vi "uTTA_Main.vi"() -> ()   [LabVIEW 2021]
uses:
  uTTA_Device_Driver/uTTA_Controls/CTL_uTTA_MeasurementStates.ctl
  uTTA_Device_Driver/uTTA_Controls/CTL_uTTA_TSP_Calibration.ctl
  uTTA_Device_Driver/uTTA_Controls/CTL_uTTA_TSP_CalStatus.ctl
  <vilib>/Utility/miscctls.llb/LVPointTypeDef.ctl
  uTTA_Device_Driver/uTTA_Controls/CTL_uTTA_PGA_Gain.ctl
  uTTA_Device_Driver/uTTA_Controls/CTL_uTTA_OperatingMode.ctl
  uTTA_Device_Driver/uTTA_Controls/CTL_uTTA_AnalogParameter.ctl
  <vilib>/Utility/error.llb/DialogType.ctl
  uTTA_Device_Driver/uTTA_SubVi/Serial_Port/uTTA_GV_Serial_Monitor.vi
panel:
  out "Progress / [%]":T1(slide)={"Numeric"=0.0, "Numeric"=3.7741935483870965, "Numeric"=2.3870967741935485} scale=0.0..100.0
  out "uTTA_CalData":T2(array[cluster])
  out "ADC Overrange":bool[](array[boolean])
  out "Heating Power":dbl format="%#_3pW"
  out "Total Runtime":timestamp=timestamp(-3599.4283056259155 s since 1904-01-01) format="%<%H:%M:%S>T"
  out "Measurement Started":timestamp=timestamp(3793474800.1504135 s since 1904-01-01) format="%<%X>T"
  out "Diode Voltages":T3(graph)
  out "Current & Temp":T4(graph)
  in  "Tab Control":T5(tab)
  out "ADC1L_Range":dbl caption="Lower Limit" format="%.2pV"
  out "ADC1H_Range":dbl caption="Upper Limit" format="%.2pV"
  in  "CH1-2 Offset":dbl(slide)=-0.4 scale=-2.5..2.5 scale format="%.2pV"
  out "ADC0H_Range1":dbl caption="Upper Limit" format="%.2pV"
  out "ADC0L_Range1":dbl caption="Lower Limit" format="%.2pV"
  out "ADC0H_Range":dbl caption="Upper Limit" format="%.2pV"
  out "ADC0L_Range":dbl caption="Lower Limit" format="%.2pV"
  in  "CH0 Offset":dbl(slide)=-0.63 scale=-2.5..2.5 scale format="%.2pV"
  in  "Sense Current":dbl(slide)=0.01 caption="CH0" min=0.0 max=0.011 step=0.0001 scale=0.0..0.011 scale format="%.1pA"
  in  "µTTA Port":refnum<visa-resource-name>="COM3"
  in  "Connect":bool
  in  "Disconnect":bool
  in  "Calibration File":path
  in  "Cooling 2":dbl=5400.0 caption="Cooling" min=60.0 max=21600.0 step=1.0 format="%#_g s"
  in  "Heating 2":dbl=5400.0 caption="Heating" min=0.0 max=10800.0 step=1.0 format="%#_g s"
  in  "Preheating":dbl=60.0 min=30.0 max=21600.0 step=1.0 format="%#_g s"
  in  "Cooling":u16(ring)=3 items=["PGA = 0", "PGA = 1", "PGA = 2", "PGA = 3"]
  in  "Heating":u16(ring) items=["PGA = 0", "PGA = 1", "PGA = 2", "PGA = 3"]
  in  "Channel Names":u16[](array[ring])=[0, 0, 0] items=["OFF", "DUMMY1", "DUMMY2", "DUMMY3", "BUZ11", "IRF1010N", "IRF1010N_M", "IRF1010N_L", "IRF1010N_R", "IRFZ44N_M", "IRFZ44N_L", "IRFZ44N_R"]
  in  "Measurement Name":string
  in  "Start":bool
  in  "Stop":bool
  in  "Test Mode":bool
  out "Measurement State":T6=enum."Cooling" caption="uTTA State"
  out "GUI State":string="EXIT"
  in  "FileManager":bool
  out "Files in Flash Memory":string[](array[string])
  in  "Autoscroll":bool
  out "Serial Monitor OUT":string
  in  "Serial Monitor":bool
  in  "Gatedriver Power":bool
  in  "Main Power supply":bool
  in  "Gatedriver":bool
  out "RunTime Error":errorcluster
  out "Exit Error":errorcluster
  out "Device Info":string
  in  "Refresh_CAL":bool
  in  "Cal_Manager":bool
  out "TSP_Channels":T7 {"Offset" format="%.3pV"; "Lin. Gain" format="%#.4pV/K"; "Quad. Gain" format="%.5pV/K²"}
  # "Measurement\nRange"
  # "Measurement Range\nHEATING        COOLING"
  # "Channel Offset"
  # "Sense Current"
  # "T I M I N G"
  # "PGA"
  # "CH0: Driver"
  # "Channel\nNames"
  # "CH1: Monitor1"
  # "CH2: Monitor 2"
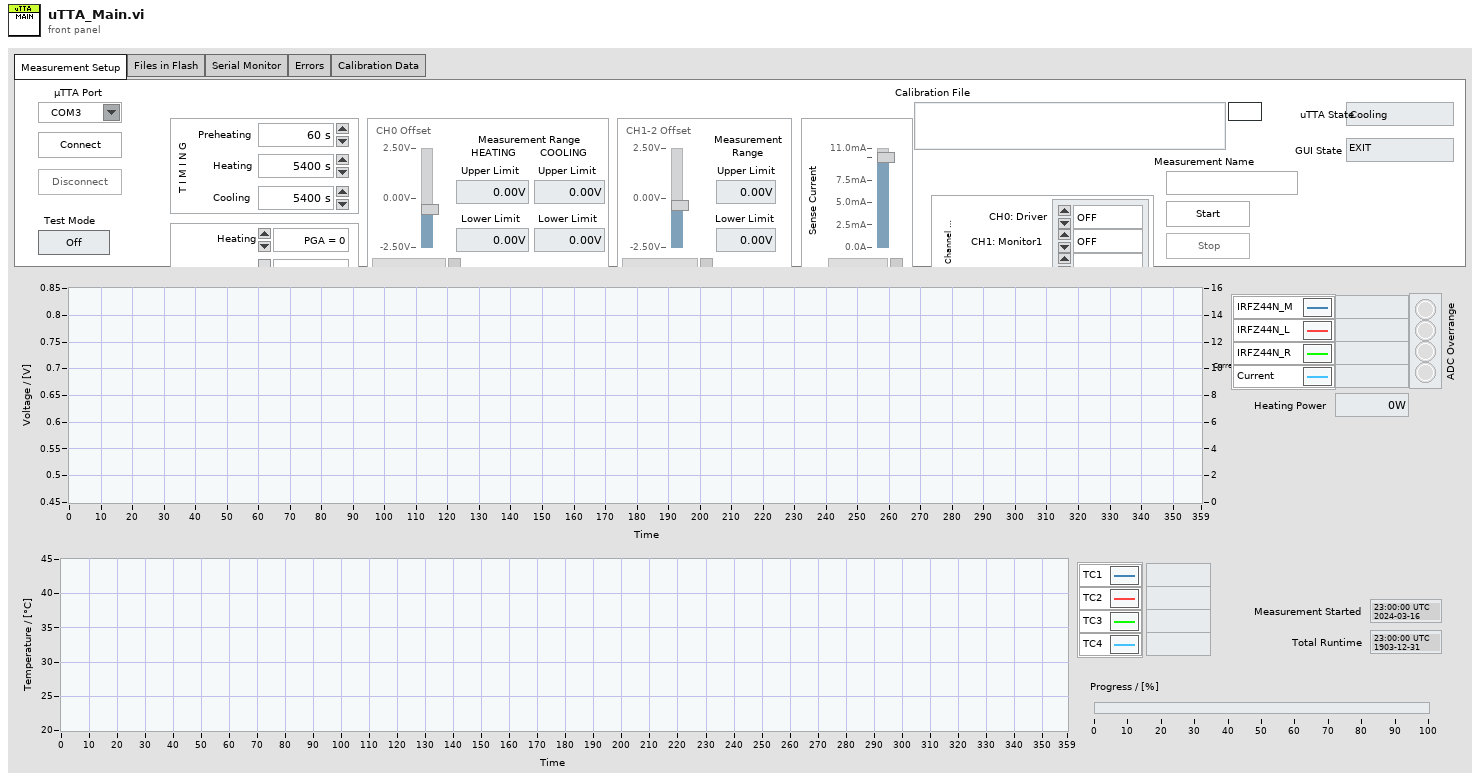
[diagram p1: front panel]
types:
  T1 = cluster{"Numeric":dbl, "Numeric":dbl, "Numeric":dbl}
  T2 = cluster{"Diff Gain":dbl, "Offset":dbl[], "Gain":dbl[]}[]
  T3 = cluster{"Diode Voltage":dbl, "Diode Voltage":dbl, "Diode Voltage":dbl, "Current":dbl}
  T4 = cluster{"Diode Voltage":dbl, "Diode Voltage":dbl, "Diode Voltage":dbl, "Diode Voltage":dbl}
  T5 = enum32{"Measurement Setup", "Files in Flash", "Serial Monitor", "Test Mode Controls", "Errors", "Calibration Data"}
  T6 = typedef "CTL_uTTA_MeasurementStates.ctl" = enum16{"Idle", "Init", "GPPowerCheck", "InitMeasFile", "Preheating", "PrepHeating", "Heating", "PrepCooling", "Cooling", "Deinit", "CloseLog", "Cal_Init", "Cal_GDPowerOn", "Cal_GDPowerCheck", "Cal_Cal", "Cal_Deinit"}
  T7 = typedef "CTL_uTTA_TSP_Calibration.ctl" = cluster{"Channel Name":string, "Offset":dbl, "Lin. Gain":dbl, "Quad. Gain":dbl, "Cal Status":T8}[]
  T8 = typedef "CTL_uTTA_TSP_CalStatus.ctl" = enum16{"Uncalibrated", "Calibrated", "Dummy"}
  T9 = typedef "LVPointTypeDef.ctl" = cluster{"Horizontal":i16, "Vertical":i16}
  T10 = typedef "CTL_uTTA_AnalogParameter.ctl" = enum16{"ISEN", "SPARE", "VOFF"}
  T11 = enum8{"Enabled", "Disabled", "Disabled and Grayed Out"}
  T12 = typedef "CTL_uTTA_PGA_Gain.ctl" = enum16{"All", "Cooling", "Heating"}
  T13 = typedef "CTL_uTTA_OperatingMode.ctl" = enum16{"NORMAL", "TEST_MODE", "TEMP_CONTROL"}
  T14 = cluster{"Diode Voltage":dbl, "Diode Voltage":dbl, "Diode Voltage":dbl, "Current":dbl}[]
  T15 = cluster{"Diode Voltage":dbl, "Diode Voltage":dbl, "Diode Voltage":dbl, "Diode Voltage":dbl}[]
  T16 = cluster{"Channel Name":string, "Offset":dbl, "Lin. Gain":dbl, "Quad. Gain":dbl, "Cal Status":T8}
  T17 = cluster{"Measurement State":T6, "Diode Voltages":dbl[], "Current":dbl, "Temperatures":dbl[], "NewData":bool, "ADC Overrange":bool[]}
  T18 = typedef "DialogType.ctl" = u16
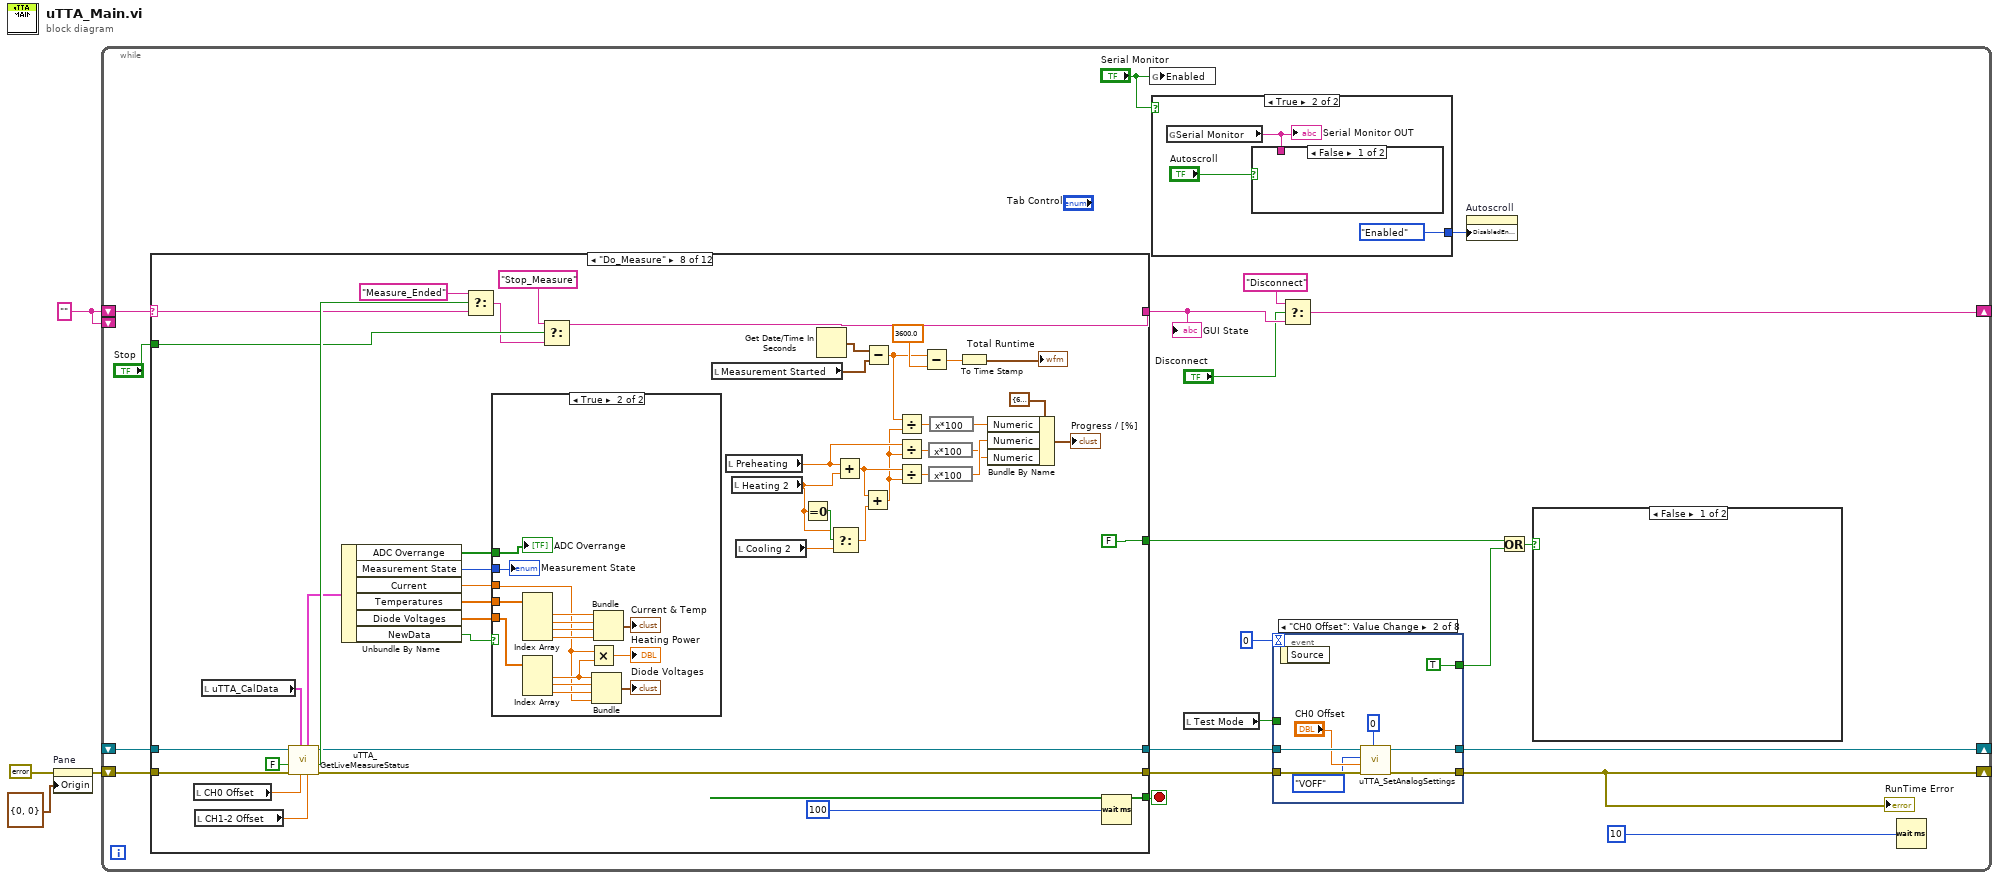
[diagram p0: block diagram]
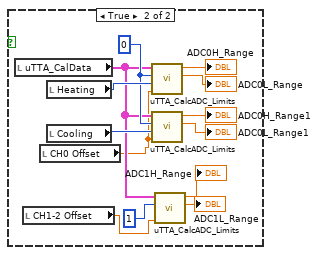
[diagram p2: hidden frame]
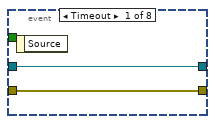
[diagram p3: hidden frame]
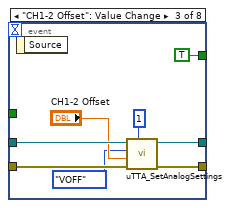
[diagram p4: hidden frame]
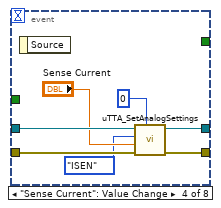
[diagram p5: hidden frame]
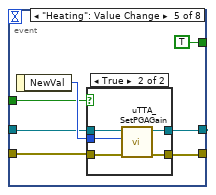
[diagram p6: hidden frame]
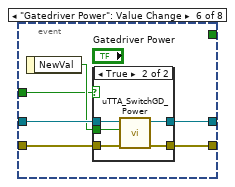
[diagram p8: hidden frame]
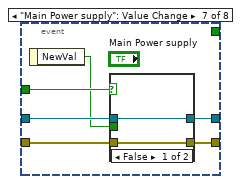
[diagram p10: hidden frame]
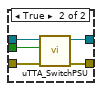
[diagram p11: hidden frame]
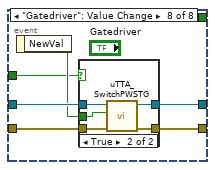
[diagram p12: hidden frame]
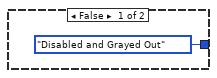
[diagram p14: hidden frame]
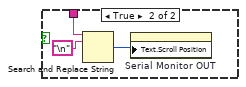
[diagram p15: hidden frame]
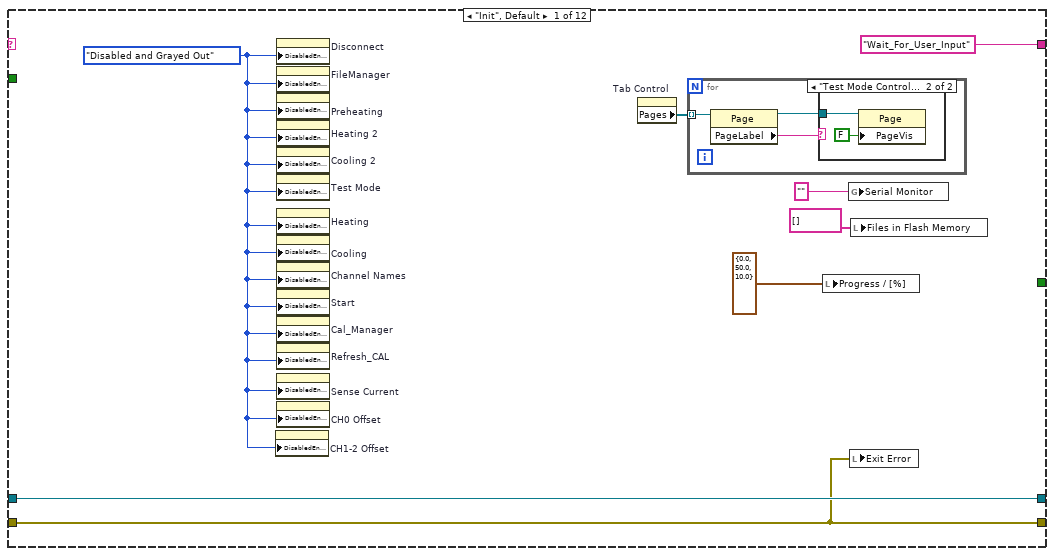
[diagram p16: hidden frame]
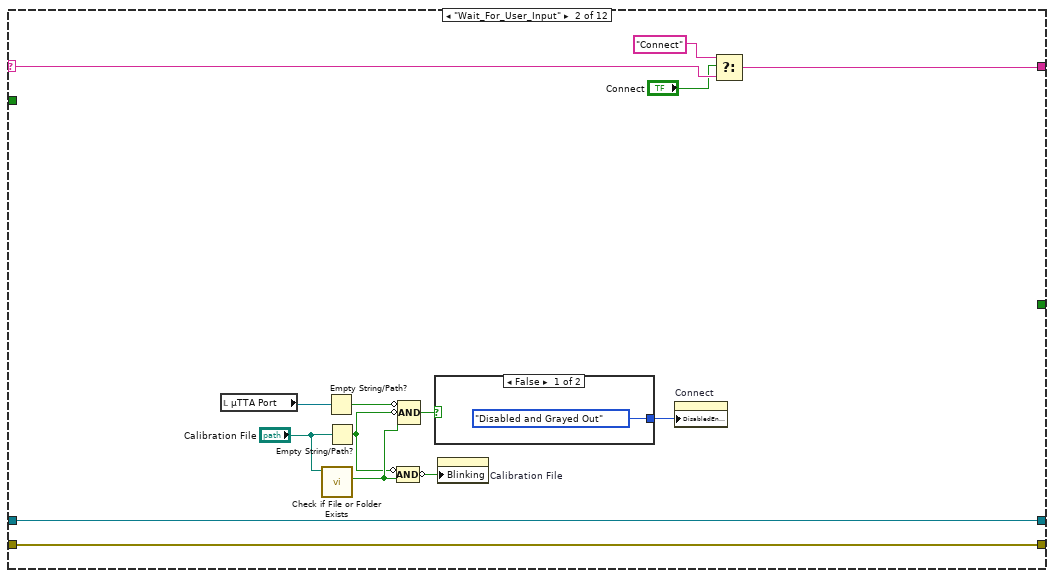
[diagram p18: hidden frame]
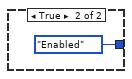
[diagram p19: hidden frame]
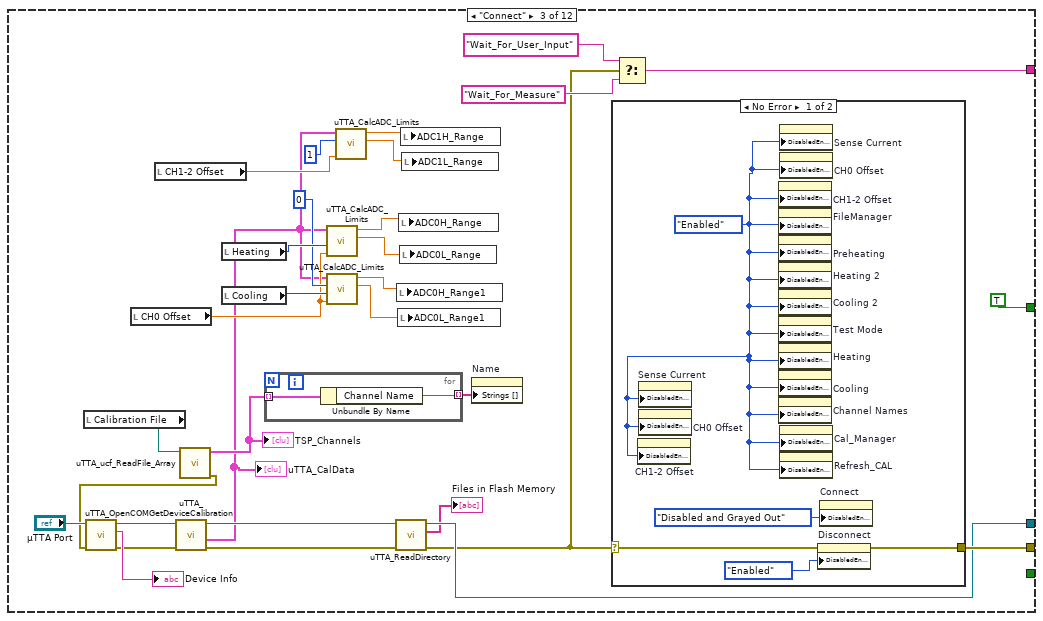
[diagram p20: hidden frame]
diagram:
  w1 = "" ("Identity")
  n1 = property on="Pane" class="Pane"(error in=errorcluster {"status"=FALSE, "code"=0, "source"=""} ("error out"), "Origin"=T9 {"Horizontal"=0, "Vertical"=0}) -> (error out=w2:errorcluster)  [unwired: 1 in, 1 out]
  n2 = while {
    shift-right: [w19] -> _
    shift-left: w1 -> [w25]
    shift-right: [w11] -> _
    shift-left: _ -> [w24]
    shift-right: [w9] -> _
    shift-left: w2 -> [w23]
    shift-left: w1 -> [_]
    stop <- w22 stop-if-true
    n3 = case shown="\"Do_Measure\"" w25 {
      selector: w25 -> [_ w149 _ w213 _ _ _ w411 _ _ _ w458]
      tunnel: ["Wait_For_User_Input" w150 w178 w212 w247 w290 "Do_Measure" ("t") w402 "Measure_Ended" ("t") "Wait_For_Measure" ("t") "EXIT" w458] -> w20
      tunnel: [w130 w147 w177 w203 w254 w296 w339 w395 w433 w438 refnum<visa-resource-name> refnum ("VISA out") w457] -> w12
      tunnel: w24 -> [w130 w147 _ w204 w253 w295 w332 w415 w435 w439 w452 w457]
      tunnel: w23 -> [w129 w146 _ w205 w252 w294 w333 w414 w434 w440 w453 w456]
      tunnel: [w129 w146 w181 w197 w249 w289 w338 w394 w432 w437 w449 w456] -> w10
      tunnel: [_ _ _ _ _ _ _ _ _ _ _ TRUE] -> w22
      tunnel: "Stop" -> [_ _ _ _ _ _ _ w405 _ _ _ _]
      tunnel: [_ _ TRUE _ _ _ _ FALSE _ _ _ _] -> w5
      frame "Init", Default {
        w125 = T11."Disabled and Grayed Out" ("Disabled")
        n4 = property on="CH1-2 Offset" class="Slide (strict)"("DisabledEnum"=w125) -> ()  [unwired: 2 in, 2 out]
        n5 = property on="Disconnect" class="Bool"("DisabledEnum"=w125) -> ()  [unwired: 2 in, 2 out]
        n6 = property on="FileManager" class="Bool"("DisabledEnum"=w125) -> ()  [unwired: 2 in, 2 out]
        n7 = property on="Preheating" class="DigNum (strict)"("DisabledEnum"=w125) -> ()  [unwired: 2 in, 2 out]
        n8 = property on="Heating 2" class="DigNum (strict)"("DisabledEnum"=w125) -> ()  [unwired: 2 in, 2 out]
        n9 = property on="Cooling 2" class="DigNum (strict)"("DisabledEnum"=w125) -> ()  [unwired: 2 in, 2 out]
        n10 = property on="Test Mode" class="Bool (strict)"("DisabledEnum"=w125) -> ()  [unwired: 2 in, 2 out]
        n11 = property on="Heating" class="Ring (strict)"("DisabledEnum"=w125) -> ()  [unwired: 2 in, 2 out]
        n12 = property on="Cooling" class="Ring (strict)"("DisabledEnum"=w125) -> ()  [unwired: 2 in, 2 out]
        n13 = property on="Channel Names" class="Arr (strict)"("DisabledEnum"=w125) -> ()  [unwired: 2 in, 2 out]
        n14 = property on="Start" class="Bool"("DisabledEnum"=w125) -> ()  [unwired: 2 in, 2 out]
        n15 = property on="Cal_Manager" class="Bool"("DisabledEnum"=w125) -> ()  [unwired: 2 in, 2 out]
        n16 = property on="Refresh_CAL" class="Bool"("DisabledEnum"=w125) -> ()  [unwired: 2 in, 2 out]
        n17 = property on="Sense Current" class="Slide (strict)"("DisabledEnum"=w125) -> ()  [unwired: 2 in, 2 out]
        n18 = property on="CH0 Offset" class="Slide (strict)"("DisabledEnum"=w125) -> ()  [unwired: 2 in, 2 out]
        n19 = property on="Tab Control" class="TabCtl (strict)"() -> ("Pages"=w127:refnum<vi>[])  [unwired: 2 in, 2 out]
        n20 = for {
          tunnel: w127 -> [w134] mode=indexing
          n21 = property class="Page"(reference=w134) -> (reference out=w132:refnum<vi>, "PageLabel"=w133:string)  [unwired: 1 in, 1 out]
          n22 = case shown="\"Test Mode Controls\"" w133 {
            tunnel: w132 -> [_ w136]
            frame "False", Default {
            }
            frame "Test Mode Controls" {
              n23 = property class="Page"(reference=w136, "PageVis"=FALSE ("Page Visible")) -> ()  [unwired: 1 in, 2 out]
            }
          }
        }
        n24 = local write "Progress / [%]"(T1 {"Numeric"=0.0, "Numeric"=50.0, "Numeric"=10.0} ("Progress")) -> ()
        n25 = global write "uTTA_GV_Serial_Monitor.vi" "Serial Monitor"("" ("Received")) -> ()
        n26 = local write "Exit Error"(w129) -> ()
        n27 = local write "Files in Flash Memory"(string[] [] ("Files in Flash Memory")) -> ()
      }
      frame "Wait_For_User_Input" {
        n28 = local read "µTTA Port"() -> (w145:refnum<visa-resource-name>)
        n29 = call <vilib>:"Check if File or Folder Exists.vi"("path"="Calibration File") -> ("file or folder exists?"=w139:bool)  [unwired: 8 in, 2 out]
        n30 = Empty String/Path?(string/path=w145) -> (empty?=w142:bool)
        n31 = Empty String/Path?(string/path="Calibration File") -> (empty?=w138:bool)
        n32 = Compound Arithmetic op=AND(invert w138, w139) -> (invert w137:bool)
        n33 = Compound Arithmetic op=AND(invert w142, invert w138, w139) -> (w141:bool)
        n34 = case shown="False" w141 {
          tunnel: [T11."Disabled and Grayed Out" ("Disabled") T11."Enabled" ("Disabled")] -> w143
          frame False {
          }
          frame True {
          }
        }
        n35 = property on="Calibration File" class="Path"("Blinking"=w137) -> ()  [unwired: 2 in, 2 out]
        n36 = property on="Connect" class="Bool"("DisabledEnum"=w143) -> ()  [unwired: 2 in, 2 out]
        n37 = Select(t="Connect", s="Connect", f=w149) -> (s? t:f=w150:string)
      }
      frame "Connect" {
        n38 = local read "Calibration File"() -> (w174:path)
        n39 = local read "CH0 Offset"() -> (w159:dbl)
        n40 = local read "CH1-2 Offset"() -> (w166:dbl)
        n41 = call "uTTA_ucf_ReadFile_Array.vi"("selected path"=w174) -> ("error out"=w173:errorcluster, "TSP_Channels"=w171:T7)  [unwired: 7 in, 2 out]
        "TSP_Channels" <- w171
        n42 = call "uTTA_OpenCOM.vi"("error in"=w173, "VISA in"="µTTA Port") -> ("error out"=w156:errorcluster, "Identity"=→"Device Info":string, "VISA out"=w157:refnum<visa-resource-name>)  [unwired: 7 in]
        n43 = call "uTTA_GetDeviceCalibration.vi"("error in"=w156, "VISA Refnum in"=w157) -> ("error out"=w154:errorcluster, "uTTA_CalData"=w153:T2, "VISA Refnum out"=w155:refnum<visa-resource-name>)  [unwired: 2 in, 1 out]
        "uTTA_CalData" <- w153
        n44 = local read "Heating"() -> (w170:u16)
        n45 = local read "Cooling"() -> (w169:u16)
        n46 = for {
          tunnel: w171 -> [w185] mode=indexing
          tunnel: [w184] -> w172 mode=indexing
          n47 = Unbundle By Name(w185) -> ("Channel Name"=w184:string)
        }
        n48 = call "uTTA_CalcADC_Limits.vi"("Offset Voltage"=w159, "PGA_Setting"=w170, "uTTA_CalData"=w153) -> ("Range Low End"=w162:dbl, "Range High End"=w163:dbl)  [unwired: 7 in]
        n49 = call "uTTA_CalcADC_Limits.vi"("Offset Voltage"=w159, "PGA_Setting"=w169, "Channel Number"=u32 0, "uTTA_CalData"=w153) -> ("Range Low End"=w160:dbl, "Range High End"=w161:dbl)  [unwired: 6 in]
        n50 = call "uTTA_CalcADC_Limits.vi"("Offset Voltage"=w166, "Channel Number"=u32 1, "uTTA_CalData"=w153) -> ("Range Low End"=w164:dbl, "Range High End"=w165:dbl)  [unwired: 7 in]
        n51 = call "uTTA_ReadDirectory.vi"("error in"=w154, "VISA Refnum in"=w155) -> ("error out"=w176:errorcluster, "Files"=→"Files in Flash Memory":string[], "VISA Refnum out"=w177:refnum<visa-resource-name>)  [unwired: 3 in]
        n52 = local write "ADC0H_Range1"(w161) -> ()
        n53 = local write "ADC0L_Range1"(w160) -> ()
        n54 = local write "ADC0H_Range"(w163) -> ()
        n55 = local write "ADC0L_Range"(w162) -> ()
        n56 = local write "ADC1H_Range"(w165) -> ()
        n57 = local write "ADC1L_Range"(w164) -> ()
        n58 = property on="Name" class="Ring (strict)"("Strings []"=w172) -> ()  [unwired: 2 in, 2 out]
        n59 = case shown="No Error" w176 {
          selector: w176 -> [w188 w191]
          tunnel: [w189 w191] -> w181
          frame No Error {
            w186 = T11."Enabled" ("Disabled")
            n60 = property on="CH1-2 Offset" class="Slide (strict)"("DisabledEnum"=w186) -> ()  [unwired: 2 in, 2 out]
            n61 = property on="Sense Current" class="Slide (strict)"("DisabledEnum"=w186) -> ()  [unwired: 2 in, 2 out]
            n62 = property on="CH0 Offset" class="Slide (strict)"("DisabledEnum"=w186) -> ()  [unwired: 2 in, 2 out]
            n63 = property on="CH1-2 Offset" class="Slide (strict)"("DisabledEnum"=w186) -> ()  [unwired: 2 in, 2 out]
            n64 = property on="FileManager" class="Bool"("DisabledEnum"=w186) -> ()  [unwired: 2 in, 2 out]
            n65 = property on="Preheating" class="DigNum (strict)"("DisabledEnum"=w186) -> ()  [unwired: 2 in, 2 out]
            n66 = property on="Heating 2" class="DigNum (strict)"("DisabledEnum"=w186) -> ()  [unwired: 2 in, 2 out]
            n67 = property on="Cooling 2" class="DigNum (strict)"("DisabledEnum"=w186) -> ()  [unwired: 2 in, 2 out]
            n68 = property on="Test Mode" class="Bool (strict)"("DisabledEnum"=w186) -> ()  [unwired: 2 in, 2 out]
            n69 = property on="Heating" class="Ring (strict)"("DisabledEnum"=w186) -> ()  [unwired: 2 in, 2 out]
            n70 = property on="Cooling" class="Ring (strict)"("DisabledEnum"=w186) -> ()  [unwired: 2 in, 2 out]
            n71 = property on="Channel Names" class="Arr (strict)"("DisabledEnum"=w186) -> ()  [unwired: 2 in, 2 out]
            n72 = property on="Sense Current" class="Slide (strict)"("DisabledEnum"=w186) -> ()  [unwired: 2 in, 2 out]
            n73 = property on="CH0 Offset" class="Slide (strict)"("DisabledEnum"=w186) -> ()  [unwired: 2 in, 2 out]
            n74 = property on="Cal_Manager" class="Bool"("DisabledEnum"=w186) -> ()  [unwired: 2 in, 2 out]
            n75 = property on="Refresh_CAL" class="Bool"("DisabledEnum"=w186) -> ()  [unwired: 2 in, 2 out]
            n76 = property on="Disconnect" class="Bool"(error in=w188, "DisabledEnum"=T11."Enabled" ("Disabled")) -> (error out=w189:errorcluster)  [unwired: 1 in, 1 out]
            n77 = property on="Connect" class="Bool"("DisabledEnum"=T11."Disabled and Grayed Out" ("Disabled")) -> ()  [unwired: 2 in, 2 out]
          }
          frame Error {
          }
        }
        n78 = Select(t="Wait_For_User_Input", s=w176, f="Wait_For_Measure" ("t")) -> (s? t:f=w178:string)
      }
      frame "Wait_For_Measure" {
        n79 = local read "Measurement Name"() -> (w216:string)
        n80 = local read "Heating 2"() -> (w194:dbl)
        n81 = case shown="True" "FileManager" {
          selector: "FileManager" -> [_ w242]
          tunnel: w204 -> [w235 w240]
          tunnel: w205 -> [w236 w243]
          tunnel: [w236 w238] -> w200
          tunnel: [w235 w239] -> w203
          frame False {
          }
          frame True {
            n82 = call "uTTA_Read_File_UI.vi"("error in"=w243, "Externally Called"=w242, "VISA resource name"=w240) -> ("error out"=w241:errorcluster)  [unwired: 4 in]
            n83 = call "uTTA_ReadDirectory.vi"("error in"=w241, "VISA Refnum in"=w240) -> ("error out"=w238:errorcluster, "Files"=w237:string[], "VISA Refnum out"=w239:refnum<visa-resource-name>)  [unwired: 3 in]
            n84 = local write "Files in Flash Memory"(w237) -> ()
          }
        }
        n85 = Greater Than 0?(x=w194) -> (x > 0?=w193:bool)
        n86 = Empty String/Path?(string/path=w216) -> (empty?=w207:bool)
        n87 = case shown="False" w193 {
          tunnel: [T11."Disabled and Grayed Out" ("Disabled") T11."Enabled" ("Disabled")] -> w192
          frame False {
          }
          frame True {
          }
        }
        n88 = property on="Measurement Name" class="Str"("Blinking"=w207) -> ()  [unwired: 2 in, 2 out]
        n89 = Compound Arithmetic op=AND(invert w207) -> (w215:bool)
        n90 = case shown="True" w215 {
          tunnel: [T11."Disabled and Grayed Out" ("Disabled") T11."Enabled" ("Disabled")] -> w214
          frame False {
          }
          frame True {
          }
        }
        n91 = property on="Cooling 2" class="DigNum (strict)"("DisabledEnum"=w192) -> ()  [unwired: 2 in, 2 out]
        n92 = property on="Heating" class="Ring (strict)"("DisabledEnum"=w192) -> ()  [unwired: 2 in, 2 out]
        n93 = case shown="True" "Refresh_CAL" {
          tunnel: w200 -> [w224 w227]
          tunnel: [w224 w226] -> w198
          frame False {
          }
          frame True {
            n94 = local read "Calibration File"() -> (w230:path)
            n95 = call "uTTA_ucf_ReadFile_Array.vi"("error in"=w227, "selected path"=w230) -> ("error out"=w226:errorcluster, "uTTA_CalData"=w225:T2, "TSP_Channels"=w228:T7)  [unwired: 6 in, 1 out]
            n96 = for {
              tunnel: w228 -> [w232] mode=indexing
              tunnel: [w231] -> w229 mode=indexing
              n97 = Unbundle By Name(w232) -> ("Channel Name"=w231:string)
            }
            n98 = local write "TSP_Channels"(w228) -> ()
            n99 = local write "uTTA_CalData"(w225) -> ()
            n100 = property on="Name" class="Ring (strict)"("Strings []"=w229) -> ()  [unwired: 2 in, 2 out]
          }
        }
        n101 = Select(t="Init_Measure_Cal", s="Test Mode", f="Init_Measure_Normal" ("t")) -> (s? t:f=w208:string)
        n102 = property on="Start" class="Bool"("DisabledEnum"=w214) -> ()  [unwired: 2 in, 2 out]
        n103 = Select(t=w208, s="Start", f=w213) -> (s? t:f=w212:string)
        n104 = case shown="True" "Start" {
          tunnel: [T11."Enabled" ("Disabled") T11."Disabled and Grayed Out" ("Disabled")] -> w199
          frame False {
          }
          frame True {
          }
        }
        n105 = local read "Calibration File"() -> (w196:path)
        n106 = property on="FileManager" class="Bool"("DisabledEnum"=w199) -> ()  [unwired: 2 in, 2 out]
        n107 = property on="Cal_Manager" class="Bool"("DisabledEnum"=w199) -> ()  [unwired: 2 in, 2 out]
        n108 = property on="Refresh_CAL" class="Bool"("DisabledEnum"=w199) -> ()  [unwired: 2 in, 2 out]
        n109 = case shown="False" "Cal_Manager" {
          selector: "Cal_Manager" -> [_ w221]
          tunnel: w198 -> [w219 w223]
          tunnel: [w219 w222] -> w197
          tunnel: w196 -> [_ w220]
          frame False {
          }
          frame True {
            n110 = call "uTTA_CreateCAL_File.vi"("error in"=w223, "Ext. called"=w221, "Ext. File Path"=w220) -> ("error out"=w222:errorcluster)  [unwired: 4 in]
          }
        }
      }
      frame "Init_Measure_Normal" {
        n111 = case shown="No Error" w252 {
          selector: w252 -> [w282 w287]
          tunnel: w253 -> [w284 w288]
          tunnel: [w285 w288] -> w251
          tunnel: [w286 w287] -> w250
          frame No Error {
            w278 = T11."Disabled and Grayed Out" ("Disabled")
            n112 = call "Time Delay9"("error in (no error)"=w282) -> ("error out"=w283:errorcluster)  [unwired: 10 in]
            n113 = property on="CH1-2 Offset" class="Slide (strict)"("DisabledEnum"=w278) -> ()  [unwired: 2 in, 2 out]
            n114 = property on="Preheating" class="DigNum (strict)"("DisabledEnum"=w278) -> ()  [unwired: 2 in, 2 out]
            n115 = property on="Heating 2" class="DigNum (strict)"("DisabledEnum"=w278) -> ()  [unwired: 2 in, 2 out]
            n116 = property on="Cooling 2" class="DigNum (strict)"("DisabledEnum"=w278) -> ()  [unwired: 2 in, 2 out]
            n117 = property on="Test Mode" class="Bool (strict)"("DisabledEnum"=w278) -> ()  [unwired: 2 in, 2 out]
            n118 = property on="Heating" class="Ring (strict)"("DisabledEnum"=w278) -> ()  [unwired: 2 in, 2 out]
            n119 = property on="Cooling" class="Ring (strict)"("DisabledEnum"=w278) -> ()  [unwired: 2 in, 2 out]
            n120 = property on="Channel Names" class="Arr (strict)"("DisabledEnum"=w278) -> ()  [unwired: 2 in, 2 out]
            n121 = property on="Sense Current" class="Slide (strict)"("DisabledEnum"=w278) -> ()  [unwired: 2 in, 2 out]
            n122 = property on="CH0 Offset" class="Slide (strict)"("DisabledEnum"=w278) -> ()  [unwired: 2 in, 2 out]
            n123 = call "uTTA_SetMode.vi"("error in"=w283, "OperatingMode"=CTL_uTTA_OperatingMode."NORMAL", "VISA Refnum in"=w284) -> ("error out"=w286:errorcluster, "VISA Refnum out"=w285:refnum<visa-resource-name>)  [unwired: 2 in, 1 out]
            n124 = property on="Start" class="Bool"("DisabledEnum"=T11."Disabled and Grayed Out" ("Disabled")) -> ()  [unwired: 2 in, 2 out]
            n125 = property on="Stop" class="Bool"("DisabledEnum"=T11."Enabled" ("Disabled")) -> ()  [unwired: 2 in, 2 out]
          }
          frame Error {
          }
        }
        n126 = call "uTTA_SetCoolingTime.vi"("error in"=w250, "CoolingTime (s)"="Cooling 2", "VISA Refnum in"=w251) -> ("error out"=w267:errorcluster, "VISA Refnum out"=w270:refnum<visa-resource-name>)  [unwired: 2 in, 1 out]
        n127 = call "Time Delay"("error in (no error)"=w267) -> ("error out"=w266:errorcluster)  [unwired: 10 in]
        n128 = call "uTTA_SetHeatingTime.vi"("error in"=w266, "HeatingTime (s)"="Heating 2", "VISA Refnum in"=w270) -> ("error out"=w265:errorcluster, "VISA Refnum out"=w269:refnum<visa-resource-name>)  [unwired: 2 in, 1 out]
        n129 = call "Time Delay2"("error in (no error)"=w265) -> ("error out"=w264:errorcluster)  [unwired: 10 in]
        n130 = call "uTTA_SetPreHeatingTime.vi"("error in"=w264, "PreHeatingTime (s)"="Preheating", "VISA Refnum in"=w269) -> ("error out"=w263:errorcluster, "VISA Refnum out"=w268:refnum<visa-resource-name>)  [unwired: 2 in, 1 out]
        n131 = call "Time Delay3"("error in (no error)"=w263) -> ("error out"=w262:errorcluster)  [unwired: 10 in]
        n132 = call "uTTA_SetPGAGain.vi"("Mode"=CTL_uTTA_PGA_Gain."Heating", "error in"=w262, "PGA Gain"="Heating", "VISA Refnum in"=w268) -> ("error out"=w261:errorcluster, "VISA Refnum out"=w273:refnum<visa-resource-name>)  [unwired: 4 in, 2 out]
        n133 = call "Time Delay4"("error in (no error)"=w261) -> ("error out"=w260:errorcluster)  [unwired: 10 in]
        n134 = call "uTTA_SetPGAGain.vi"("Mode"=CTL_uTTA_PGA_Gain."Cooling", "error in"=w260, "PGA Gain"="Cooling", "VISA Refnum in"=w273) -> ("error out"=w258:errorcluster, "VISA Refnum out"=w272:refnum<visa-resource-name>)  [unwired: 4 in, 2 out]
        n135 = call "Time Delay5"("error in (no error)"=w258) -> ("error out"=w259:errorcluster)  [unwired: 10 in]
        n136 = call "uTTA_SetDUT_Name.vi"("error in"=w259, "DUT Name"="Measurement Name", "VISA Refnum in"=w272) -> ("error out"=w249:errorcluster, "VISA Refnum out"=w254:refnum<visa-resource-name>)  [unwired: 6 in, 1 out]
        n137 = Select(t="Measure_Ended", s=w249, f="Init_Measure" ("t")) -> (s? t:f=w247:string)
      }
      frame "Init_Measure_Cal" {
        n138 = case shown="No Error" w294 {
          selector: w294 -> [w308 w312]
          tunnel: w295 -> [w304 w313]
          tunnel: [w306 w313] -> w296
          tunnel: [w305 w312] -> w289
          frame No Error {
            w303 = T11."Disabled and Grayed Out" ("Disabled")
            w302 = T11."Enabled" ("Disabled")
            n139 = call "Time Delay17"("error in (no error)"=w308) -> ("error out"=w309:errorcluster)  [unwired: 10 in]
            n140 = call "uTTA_SetMode.vi"("error in"=w309, "OperatingMode"=CTL_uTTA_OperatingMode."TEST_MODE" ("t"), "VISA Refnum in"=w304) -> ("error out"=w310:errorcluster, "VISA Refnum out"=w306:refnum<visa-resource-name>)  [unwired: 2 in, 1 out]
            n141 = property on="Main Power supply" class="Bool (strict)"("DisabledEnum"=w302) -> ()  [unwired: 2 in, 2 out]
            n142 = property on="Gatedriver Power" class="Bool (strict)"("DisabledEnum"=w302) -> ()  [unwired: 2 in, 2 out]
            n143 = property on="Preheating" class="DigNum (strict)"("DisabledEnum"=w303) -> ()  [unwired: 2 in, 2 out]
            n144 = property on="Heating 2" class="DigNum (strict)"("DisabledEnum"=w303) -> ()  [unwired: 2 in, 2 out]
            n145 = property on="Cooling 2" class="DigNum (strict)"("DisabledEnum"=w303) -> ()  [unwired: 2 in, 2 out]
            n146 = property on="Test Mode" class="Bool (strict)"("DisabledEnum"=w303) -> ()  [unwired: 2 in, 2 out]
            n147 = property on="Cooling" class="Ring (strict)"("DisabledEnum"=w303) -> ()  [unwired: 2 in, 2 out]
            n148 = property on="Channel Names" class="Arr (strict)"("DisabledEnum"=w303) -> ()  [unwired: 2 in, 2 out]
            n149 = property on="Gatedriver" class="Bool (strict)"("DisabledEnum"=w302) -> ()  [unwired: 2 in, 2 out]
            n150 = property on="Heating" class="Ring (strict)"("DisabledEnum"=w302) -> ()  [unwired: 2 in, 2 out]
            n151 = call "Time Delay18"("error in (no error)"=w310) -> ("error out"=w305:errorcluster)  [unwired: 10 in]
            n152 = property on="Start" class="Bool"("DisabledEnum"=T11."Disabled and Grayed Out" ("Disabled")) -> ()  [unwired: 2 in, 2 out]
            n153 = property on="Stop" class="Bool"("DisabledEnum"=w302) -> ()  [unwired: 2 in, 2 out]
          }
          frame Error {
          }
        }
        n154 = property on="Tab Control" class="TabCtl (strict)"() -> ("Pages"=w293:refnum<vi>[])  [unwired: 2 in, 2 out]
        n155 = for {
          tunnel: w293 -> [w299] mode=indexing
          n156 = property class="Page"(reference=w299) -> (reference out=w297:refnum<vi>, "PageLabel"=w298:string)  [unwired: 1 in, 1 out]
          n157 = case shown="\"Test Mode Controls\"" w298 {
            tunnel: w297 -> [_ w301]
            frame "False", Default {
            }
            frame "Test Mode Controls" {
              n158 = property class="Page"(reference=w301, "PageVis"=TRUE ("Page Visible")) -> ()  [unwired: 1 in, 2 out]
            }
          }
        }
        n159 = Select(t="Measure_Ended", s=w289, f="Init_Measure" ("t")) -> (s? t:f=w290:string)
      }
      frame "Init_Measure" {
        w316 = CTL_uTTA_AnalogParameter."VOFF" ("Parameter")
        n160 = local read "TSP_Channels"() -> (w334:T7)
        n161 = for {
          shift-right: [w348] -> w328
          shift-left: w332 -> [w349]
          shift-right: [w347] -> w329
          shift-left: w333 -> [w345]
          tunnel: "Channel Names" -> [w343] mode=indexing
          tunnel: w334 -> [w344]
          i -> [w346]
          n162 = Index Array(array=w344, index=w343) -> (element=w342:T16)
          n163 = Unbundle By Name(w342) -> ("Channel Name"=w340:string)
          n164 = String Length(string=w340) -> (length=w341:i32)
          n165 = case shown="1.." w341 {
            tunnel: w349 -> [w351 w362]
            tunnel: [w351 w361] -> w348
            tunnel: [w350 w360] -> w347
            tunnel: w346 -> [_ w355]
            tunnel: w345 -> [w350 w358]
            tunnel: w342 -> [_ w356]
            tunnel: w340 -> [_ w354]
            frame 0, Default {
            }
            frame 1.. {
              n166 = call "Time Delay6"("error in (no error)"=w358) -> ("error out"=w359:errorcluster)  [unwired: 10 in]
              n167 = Increment(x=w355) -> (x+1=w357:i32)
              n168 = Not Equal?(x=w354, y="OFF") -> (x != y?=w352:bool)
              n169 = call "uTTA_SetCH_Description.vi"("error in"=w359, "Channel No"=w357, "Channel Description"=w356, "VISA Refnum in"=w362) -> ("error out"=w360:errorcluster, "VISA Refnum out"=w361:refnum<visa-resource-name>)  [unwired: 1 in, 1 out]
              n170 = property on="Diode Voltages" class="WFChart (strict)"("Active Plot"=w355, "Plot.Plot Name"=w354, "Plot.Visible?"=w352) -> ()  [unwired: 2 in, 2 out]
            }
          }
        }
        n171 = Get Date/Time In Seconds() -> (seconds since 1Jan1904=→"Measurement Started":timestamp)
        n172 = property on="Current & Temp" class="WFChart (strict)"("History Data"=T15 []) -> ()  [unwired: 2 in, 2 out]
        n173 = property on="Diode Voltages" class="WFChart (strict)"("History Data"=T14 []) -> ()  [unwired: 2 in, 2 out]
        n174 = local read "Sense Current"() -> (w320:dbl)
        n175 = local read "CH0 Offset"() -> (w321:dbl)
        n176 = local read "CH1-2 Offset"() -> (w319:dbl)
        n177 = call "uTTA_SetAnalogSettings.vi"("Number"=u32 0, "error in"=w329, "Set Value"=w320, "Parameter"=CTL_uTTA_AnalogParameter."ISEN", "VISA Refnum in"=w328) -> ("error out"=w327:errorcluster, "VISA Refnum out"=w326:refnum<visa-resource-name>)  [unwired: 2 in, 1 out]
        n178 = call "uTTA_SetAnalogSettings.vi"("Number"=u32 0, "error in"=w327, "Set Value"=w321, "Parameter"=w316, "VISA Refnum in"=w326) -> ("error out"=w325:errorcluster, "VISA Refnum out"=w324:refnum<visa-resource-name>)  [unwired: 2 in, 1 out]
        n179 = call "uTTA_SetAnalogSettings.vi"("Number"=u32 1, "error in"=w325, "Set Value"=w319, "Parameter"=w316, "VISA Refnum in"=w324) -> ("error out"=w322:errorcluster, "VISA Refnum out"=w323:refnum<visa-resource-name>)  [unwired: 2 in, 1 out]
        n180 = case shown="No Error" w322 {
          selector: w322 -> [w364 w369]
          tunnel: w323 -> [w363 w370]
          tunnel: [w368 w370] -> w339
          tunnel: [w367 w369] -> w338
          frame No Error {
            n181 = call "Time Delay8"("error in (no error)"=w364) -> ("error out"=w365:errorcluster)  [unwired: 10 in]
            n182 = call "uTTA_SetMeasure.vi"("error in"=w365, "Action"=enum16{"STOP", "START"}."START", "VISA Refnum in"=w363) -> ("error out"=w367:errorcluster, "VISA Refnum out"=w368:refnum<visa-resource-name>)  [unwired: 2 in, 1 out]
          }
          frame Error {
          }
        }
      }
      frame "Do_Measure" {
        n183 = local read "CH0 Offset"() -> (w392:dbl)
        n184 = local read "CH1-2 Offset"() -> (w391:dbl)
        n185 = local read "uTTA_CalData"() -> (w393:T2)
        n186 = call "uTTA_GetLiveMeasureStatus.vi"("CH1&2 Offset Voltage"=w391, "CH0 Offset Voltage"=w392, "uTTA_CalData"=w393, "error in"=w414, "CalibrationMode"=FALSE, "VISA Refnum in"=w415) -> ("error out"=w394:errorcluster, "Measurement Completed"=w413:bool, "VISA Refnum out"=w395:refnum<visa-resource-name>, "Measurement Data"=w410:T17)  [unwired: 1 in, 1 out]
        n187 = Unbundle By Name(w410) -> ("ADC Overrange"=w396:bool[], "Measurement State"=w409:T6, "Current"=w408:dbl, "Temperatures"=w407:dbl[], "Diode Voltages"=w406:dbl[], "NewData"=w401:bool)
        n188 = Select(t="Measure_Ended", s=w413, f=w411) -> (s? t:f=w404:string)
        n189 = case shown="True" w401 {
          tunnel: w409 -> [_ w430]
          tunnel: w408 -> [_ w417]
          tunnel: w407 -> [_ w423]
          tunnel: w406 -> [_ w421]
          tunnel: w396 -> [_ w416]
          frame False {
          }
          frame True {
            n190 = Index Array(array=w423) -> (element #1=w428:dbl, element #2=w427:dbl, element #3=w426:dbl, element #4=w425:dbl)  [unwired: 4 in]
            n191 = Index Array(array=w421) -> (element #1=w420:dbl, element #2=w419:dbl, element #3=w418:dbl)  [unwired: 3 in]
            n192 = Multiply(x=w417, y=w420) -> (x*y=→"Heating Power":dbl)
            n193 = Bundle("Diode Voltage"=w420, "Diode Voltage"=w419, "Diode Voltage"=w418, "Current"=w417) -> (→"Diode Voltages":T3)  [unwired: 1 in]
            n194 = Bundle("Diode Voltage"=w428, "Diode Voltage"=w427, "Diode Voltage"=w426, "Diode Voltage"=w425) -> (→"Current & Temp":T4)  [unwired: 1 in]
            "Measurement State" <- w430
            "ADC Overrange" <- w416
          }
        }
        n195 = Select(t="Stop_Measure", s=w405, f=w404) -> (s? t:f=w402:string)
        n196 = local read "Measurement Started"() -> (w387:timestamp)
        n197 = local read "Preheating"() -> (w386:dbl)
        n198 = local read "Heating 2"() -> (w371:dbl)
        n199 = local read "Cooling 2"() -> (w373:dbl)
        n200 = Equal To 0?(x=w371) -> (x = 0?=w374:bool)
        n201 = Get Date/Time In Seconds() -> (seconds since 1Jan1904=w397:timestamp)
        n202 = Select(t=w371, s=w374, f=w373) -> (s? t:f=w372:dbl)
        n203 = Add(x=w386, y=w371) -> (x+y=w384:dbl)
        n204 = Add(x=w384, y=w372) -> (x+y=w383:dbl)
        n205 = Subtract(x=w397, y=w387) -> (x-y=w385:dbl)
        n206 = Divide(x=w385, y=w383) -> (x/y=w382:dbl)
        n207 = Divide(x=w386, y=w383) -> (x/y=w381:dbl)
        n208 = Divide(x=w384, y=w383) -> (x/y=w380:dbl)
        n209 = Subtract(x=w385, y=3600.0) -> (x-y=w399:dbl)
        n210 = expression code="x*100"(w381) -> (w375:dbl)
        n211 = expression code="x*100"(w380) -> (w377:dbl)
        n212 = expression code="x*100"(w382) -> (w376:dbl)
        n213 = To Time Stamp(1:w399) -> (0:→"Total Runtime":timestamp)
        n214 = Bundle By Name(cluster=T1 {"Numeric"=60.96774193548387, "Numeric"=33.87096774193548, "Numeric"=81.61290322580645} ("Progress"), "Numeric"=w376, "Numeric"=w377, "Numeric"=w375) -> (→"Progress / [%]":T1)
        n215 = Wait (ms)(milliseconds to wait=u32 100) -> ()  [unwired: 1 out]
      }
      frame "Stop_Measure" {
        n216 = call "uTTA_SetMeasure.vi"("error in"=w434, "Action"=enum16{"STOP", "START"}."STOP", "VISA Refnum in"=w435) -> ("error out"=w432:errorcluster, "VISA Refnum out"=w433:refnum<visa-resource-name>)  [unwired: 2 in, 1 out]
      }
      frame "Measure_Ended" {
        w442 = T11."Enabled" ("Disabled")
        n217 = call "uTTA_ReadDirectory.vi"("error in"=w440, "VISA Refnum in"=w439) -> ("error out"=w437:errorcluster, "Files"=w441:string[], "VISA Refnum out"=w438:refnum<visa-resource-name>)  [unwired: 3 in]
        n218 = local write "Files in Flash Memory"(w441) -> ()
        n219 = property on="FileManager" class="Bool"("DisabledEnum"=w442) -> ()  [unwired: 2 in, 2 out]
        n220 = property on="Preheating" class="DigNum (strict)"("DisabledEnum"=w442) -> ()  [unwired: 2 in, 2 out]
        n221 = property on="Heating 2" class="DigNum (strict)"("DisabledEnum"=w442) -> ()  [unwired: 2 in, 2 out]
        n222 = property on="Cooling 2" class="DigNum (strict)"("DisabledEnum"=w442) -> ()  [unwired: 2 in, 2 out]
        n223 = property on="Test Mode" class="Bool (strict)"("DisabledEnum"=w442) -> ()  [unwired: 2 in, 2 out]
        n224 = property on="Heating" class="Ring (strict)"("DisabledEnum"=w442) -> ()  [unwired: 2 in, 2 out]
        n225 = property on="Cooling" class="Ring (strict)"("DisabledEnum"=w442) -> ()  [unwired: 2 in, 2 out]
        n226 = property on="Channel Names" class="Arr (strict)"("DisabledEnum"=w442) -> ()  [unwired: 2 in, 2 out]
        n227 = property on="Cal_Manager" class="Bool"("DisabledEnum"=w442) -> ()  [unwired: 2 in, 2 out]
        n228 = property on="Refresh_CAL" class="Bool"("DisabledEnum"=w442) -> ()  [unwired: 2 in, 2 out]
        n229 = property on="Start" class="Bool"("DisabledEnum"=T11."Enabled" ("Disabled")) -> ()  [unwired: 2 in, 2 out]
        n230 = property on="Stop" class="Bool"("DisabledEnum"=T11."Disabled and Grayed Out" ("Disabled")) -> ()  [unwired: 2 in, 2 out]
      }
      frame "Disconnect" {
        w448 = T18 0 items=["no dialog", "OK message", "continue or stop message", "OK message + warnings", "continue/stop + warnings"] ("type of dialog (OK msg:1)")
        n231 = VISA Close(VISA resource name=w452, error in (no error)=w453) -> (error out=w446:errorcluster)
        "Exit Error" <- w446
        n232 = property on="Connect" class="Bool"("DisabledEnum"=T11."Enabled" ("Disabled")) -> ()  [unwired: 2 in, 2 out]
        n233 = property on="Disconnect" class="Bool"("DisabledEnum"=T11."Disabled and Grayed Out" ("Disabled")) -> ()  [unwired: 2 in, 2 out]
        n234 = call <vilib>:"Simple Error Handler.vi"("type of dialog (OK msg:1)"=w448, "error in (no error)"=w446) -> ("error out"=w449:errorcluster)  [unwired: 3 in, 4 out]
      }
      frame "EXIT" {
      }
    }
    "GUI State" <- w20
    n235 = global write "uTTA_GV_Serial_Monitor.vi" "Enabled"("Serial Monitor") -> ()
    n236 = case shown="True" "Serial Monitor" {
      tunnel: [T11."Disabled and Grayed Out" ("Disabled") T11."Enabled" ("Disabled")] -> w15
      frame False {
      }
      frame True {
        n237 = global read "uTTA_GV_Serial_Monitor.vi" "Serial Monitor"() -> (w120:string)
        "Serial Monitor OUT" <- w120
        n238 = case shown="False" "Autoscroll" {
          tunnel: w120 -> [_ w123]
          frame False {
          }
          frame True {
            n239 = Search and Replace String(input string=w123, search string="\n") -> (number of replacements=w121:i32)  [unwired: 6 in, 3 out]
            n240 = property on="Serial Monitor OUT" class="Str"("Text.Scroll Position"=w121) -> ()  [unwired: 2 in, 2 out]
          }
        }
      }
    }
    n241 = local read "Test Mode"() -> (w8:bool)
    n242 = event shown="[1] \"CH0 Offset\": Value Change" {
      selector: _ -> [_ _ _ _ _ _ _ _]
      dyn-events: _ -> [_ _ _ _ _ _ _ _]
      timeout: 0 -> [_ _ _ _ _ _ _ _]
      tunnel: w12 -> [w40 w48 w56 w63 w68 w83 w96 w109]
      tunnel: w10 -> [w39 w47 w55 w62 w66 w82 w95 w106]
      tunnel: [w40 w46 w54 w61 w67 w81 w94 w108] -> w11
      tunnel: [w39 w45 w53 w60 w65 w80 w93 w107] -> w9
      tunnel: w8 -> [_ _ _ _ w69 w78 w92 w104]
      tunnel: [_ TRUE TRUE _ TRUE _ _ _] -> w6
      event Timeout {
        n243 = event-data() -> ()  [unwired: 1 in, 1 out]
      }
      event "CH0 Offset": Value Change {
        n244 = event-data() -> ()  [unwired: 1 in, 1 out]
        n245 = call "uTTA_SetAnalogSettings.vi"("Number"=u32 0, "error in"=w47, "Set Value"="CH0 Offset", "Parameter"=CTL_uTTA_AnalogParameter."VOFF", "VISA Refnum in"=w48) -> ("error out"=w45:errorcluster, "VISA Refnum out"=w46:refnum<visa-resource-name>)  [unwired: 2 in, 1 out]
      }
      event "CH1-2 Offset": Value Change {
        n246 = event-data() -> ()  [unwired: 1 in, 1 out]
        n247 = call "uTTA_SetAnalogSettings.vi"("Number"=u32 1, "error in"=w55, "Set Value"="CH1-2 Offset", "Parameter"=CTL_uTTA_AnalogParameter."VOFF", "VISA Refnum in"=w56) -> ("error out"=w53:errorcluster, "VISA Refnum out"=w54:refnum<visa-resource-name>)  [unwired: 2 in, 1 out]
      }
      event "Sense Current": Value Change {
        n248 = event-data() -> ()  [unwired: 1 in, 1 out]
        n249 = call "uTTA_SetAnalogSettings.vi"("Number"=u32 0, "error in"=w62, "Set Value"="Sense Current", "Parameter"=CTL_uTTA_AnalogParameter."ISEN", "VISA Refnum in"=w63) -> ("error out"=w60:errorcluster, "VISA Refnum out"=w61:refnum<visa-resource-name>)  [unwired: 2 in, 1 out]
      }
      event "Heating": Value Change {
        n250 = event-data() -> ("NewVal"=w70:u16)  [unwired: 1 in]
        n251 = case shown="True" w69 {
          tunnel: w66 -> [w71 w77]
          tunnel: w68 -> [w72 w76]
          tunnel: [w72 w75] -> w67
          tunnel: [w71 w74] -> w65
          tunnel: w70 -> [_ w73]
          frame False {
          }
          frame True {
            n252 = call "uTTA_SetPGAGain.vi"("error in"=w77, "PGA Gain"=w73, "VISA Refnum in"=w76) -> ("error out"=w74:errorcluster, "VISA Refnum out"=w75:refnum<visa-resource-name>)  [unwired: 5 in, 2 out]
          }
        }
      }
      event "Gatedriver Power": Value Change {
        n253 = event-data() -> ("NewVal"=w79:bool)  [unwired: 1 in]
        n254 = case shown="True" w78 {
          tunnel: w83 -> [w85 w90]
          tunnel: w82 -> [w84 w89]
          tunnel: [w85 w88] -> w81
          tunnel: [w84 w87] -> w80
          tunnel: w79 -> [_ w86]
          frame False {
          }
          frame True {
            n255 = call "uTTA_SwitchGD_Power.vi"("error in"=w89, "GD Power Enable"=w86, "VISA Refnum in"=w90) -> ("error out"=w87:errorcluster, "VISA Refnum out"=w88:refnum<visa-resource-name>)  [unwired: 2 in, 1 out]
          }
        }
      }
      event "Main Power supply": Value Change {
        n256 = event-data() -> ("NewVal"=w91:bool)  [unwired: 1 in]
        n257 = case shown="False" w92 {
          tunnel: w96 -> [w98 w103]
          tunnel: w95 -> [w97 w102]
          tunnel: [w98 w101] -> w94
          tunnel: [w97 w100] -> w93
          tunnel: w91 -> [_ w99]
          frame False {
          }
          frame True {
            n258 = call "uTTA_SwitchPSU.vi"("error in"=w102, "PSU Enable"=w99, "VISA Refnum in"=w103) -> ("error out"=w100:errorcluster, "VISA Refnum out"=w101:refnum<visa-resource-name>)  [unwired: 2 in, 1 out]
          }
        }
      }
      event "Gatedriver": Value Change {
        n259 = event-data() -> ("NewVal"=w105:bool)  [unwired: 1 in]
        n260 = case shown="True" w104 {
          tunnel: w109 -> [w111 w116]
          tunnel: [w111 w115] -> w108
          tunnel: [w110 w114] -> w107
          tunnel: w106 -> [w110 w113]
          tunnel: w105 -> [_ w112]
          frame False {
          }
          frame True {
            n261 = call "uTTA_SwitchPWSTG.vi"("error in"=w113, "Powerstage Enable"=w112, "VISA Refnum in"=w116) -> ("error out"=w114:errorcluster, "VISA Refnum out"=w115:refnum<visa-resource-name>)  [unwired: 2 in, 1 out]
          }
        }
      }
    }
    "RunTime Error" <- w9
    n262 = Select(t="Disconnect", s="Disconnect", f=w20) -> (s? t:f=w19:string)
    n263 = property on="Autoscroll" class="Bool (strict)"("DisabledEnum"=w15) -> ()  [unwired: 2 in, 2 out]
    n264 = Or(x=w5, y=w6) -> (x .or. y?=w7:bool)
    n265 = case shown="False" w7 {
      frame False {
      }
      frame True {
        w29 = u32 0 ("Channel Number")
        n266 = local read "uTTA_CalData"() -> (w28:T2)
        n267 = local read "CH1-2 Offset"() -> (w27:dbl)
        n268 = local read "CH0 Offset"() -> (w26:dbl)
        n269 = local read "Heating"() -> (w30:u16)
        n270 = local read "Cooling"() -> (w31:u16)
        n271 = call "uTTA_CalcADC_Limits.vi"("Offset Voltage"=w26, "PGA_Setting"=w30, "Channel Number"=w29, "uTTA_CalData"=w28) -> ("Range Low End"=→"ADC0L_Range":dbl, "Range High End"=→"ADC0H_Range":dbl)  [unwired: 6 in]
        n272 = call "uTTA_CalcADC_Limits.vi"("Offset Voltage"=w26, "PGA_Setting"=w31, "Channel Number"=w29, "uTTA_CalData"=w28) -> ("Range Low End"=→"ADC0L_Range1":dbl, "Range High End"=→"ADC0H_Range1":dbl)  [unwired: 6 in]
        n273 = call "uTTA_CalcADC_Limits.vi"("Offset Voltage"=w27, "Channel Number"=u32 1, "uTTA_CalData"=w28) -> ("Range Low End"=→"ADC1L_Range":dbl, "Range High End"=→"ADC1H_Range":dbl)  [unwired: 7 in]
      }
    }
    n274 = Wait (ms)(milliseconds to wait=u32 10) -> ()  [unwired: 1 out]
  }
